vi "sync item to string type.vi"(11 "sync item":T1) -> (2 "variable name":string, 3 "variable type":string)   [LabVIEW 2013, in "Shared Memory editor node.lvclass"]
uses:
  Shared Memory editor node.lvclass
  sync/sync item.ctl
  sync/sync mechanism.ctl
  module/configuration/Shared Memory configuration.lvclass
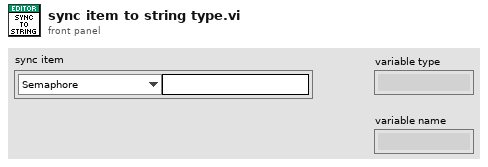
[diagram p1: front panel]
types:
  T1 = typedef "Shared Memory configuration.lvclass/sync item.ctl" = cluster{"mechanism":T2, "name":string}
  T2 = typedef "Shared Memory configuration.lvclass/sync mechanism.ctl" = enum16{"Semaphore"}
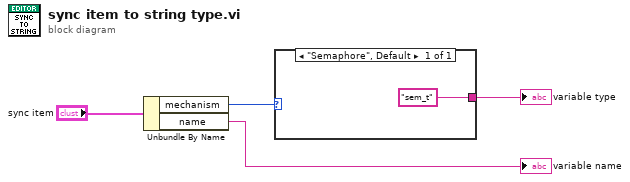
[diagram p0: block diagram]
diagram:
  n1 = Unbundle By Name("sync item") -> ("mechanism"=w3:T2, "name"=→"variable name":string)
  n2 = case shown="\"Semaphore\", Default" w3 {
    tunnel: ["sem_t"] -> w2
    frame "Semaphore", Default {
    }
  }
  "variable type" <- w2
